vi "Write WebBrowser_ActiveX.vi"(8 "error in (no error)":errorcluster, 10 "WebBrowser_ActiveX":refnum<k7>, 11 "WebBrowser_Mgmt in":refnum<class "WebBrowser_Mgmt.lvclass">) -> (0 "error out":errorcluster, 3 "WebBrowser_Mgmt out":refnum<class "WebBrowser_Mgmt.lvclass">)   [LabVIEW 2016, in "WebBrowser_Mgmt.lvclass"]
uses:
  WebBrowser_Mgmt.lvclass
  WebBrowser_Mgmt.lvclass/WebBrowser_Mgmt.ctl
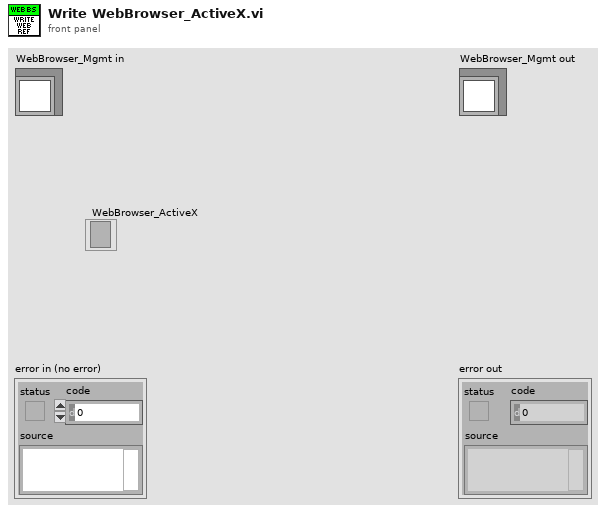
[diagram p1: front panel]
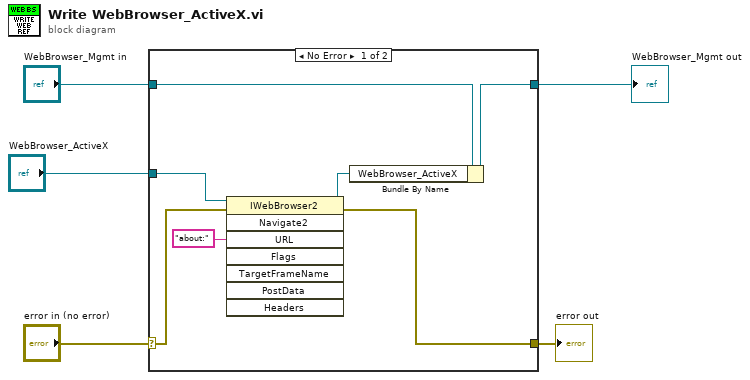
[diagram p0: block diagram]
diagram:
  n1 = case shown="No Error" "error in (no error)" {
    selector: "error in (no error)" -> [w9 w13]
    tunnel: [w8 w13] -> w4
    tunnel: [w11 w14] -> w2
    tunnel: "WebBrowser_Mgmt in" -> [w12 w14]
    tunnel: "WebBrowser_ActiveX" -> [w7 _]
    frame No Error {
      n2 = invoke class="IWebBrowser2" method="Navigate2"(reference=w7, error in=w9, "URL"="about:") -> (reference out=w6:refnum<k7>, error out=w8:errorcluster)  [unwired: 5 in, 6 out]
      n3 = Bundle By Name(cluster=w12, "WebBrowser_ActiveX"=w6) -> (w11:refnum<class "WebBrowser_Mgmt.lvclass">)
    }
    frame Error {
    }
  }
  "error out" <- w4
  "WebBrowser_Mgmt out" <- w2
